vi "Assignment #4 Sarah Bailey.vi"(11 "SCROLLING TEXT":string="LabVIEW VI Assignment ") -> (3 "Array":bool[][](array[boolean])=[[FALSE, FALSE, FALSE, FALSE, TRUE, TRUE, TRUE, FALSE, FALSE, FALSE, FALSE, TRUE, TRUE, TRUE, FALSE, FALSE, FALSE, FALSE, TRUE, TRUE, TRUE, FALSE, FALSE, FALSE, TRUE, TRUE, TRUE, TRUE, TRUE, FALSE, FALSE, FALSE, TRUE, TRUE, TRUE, TRUE, FALSE, FALSE, TRUE, FALSE, FALSE, FALSE, TRUE, FALSE, FALSE, TRUE, FALSE, FALSE, FALSE, TRUE, FALSE, FALSE, TRUE, TRUE, TRUE, TRUE, TRUE, FALSE, FALSE, TRUE, FALSE, FALSE, FALSE, TRUE, FALSE, FALSE, TRUE, TRUE, TRUE], [FALSE, FALSE, FALSE, TRUE, FALSE, FALSE, FALSE, TRUE, FALSE, FALSE, TRUE, FALSE, FALSE, FALSE, TRUE, FALSE, FALSE, TRUE, FALSE, FALSE, FALSE, TRUE, FALSE, FALSE, FALSE, FALSE, TRUE, FALSE, FALSE, FALSE, FALSE, TRUE, FALSE, FALSE, FALSE, FALSE, FALSE, FALSE, TRUE, TRUE, FALSE, FALSE, TRUE, FALSE, FALSE, TRUE, TRUE, FALSE, TRUE, TRUE, FALSE, FALSE, TRUE, FALSE, FALSE, FALSE, FALSE, FALSE, FALSE, TRUE, TRUE, FALSE, FALSE, TRUE, FALSE, FALSE, FALSE, FALSE, TRUE], [FALSE, FALSE, FALSE, TRUE, FALSE, FALSE, FALSE, TRUE, FALSE, FALSE, TRUE, FALSE, FALSE, FALSE, FALSE, FALSE, FALSE, TRUE, FALSE, FALSE, FALSE, FALSE, FALSE, FALSE, FALSE, FALSE, TRUE, FALSE, FALSE, FALSE, FALSE, TRUE, FALSE, FALSE, FALSE, FALSE, FALSE, FALSE, TRUE, FALSE, TRUE, FALSE, TRUE, FALSE, FALSE, TRUE, FALSE, TRUE, FALSE, TRUE, FALSE, FALSE, TRUE, FALSE, FALSE, FALSE, FALSE, FALSE, FALSE, TRUE, FALSE, TRUE, FALSE, TRUE, FALSE, FALSE, FALSE, FALSE, TRUE], [FALSE, FALSE, FALSE, TRUE, TRUE, TRUE, TRUE, TRUE, FALSE, FALSE, FALSE, TRUE, TRUE, TRUE, FALSE, FALSE, FALSE, FALSE, TRUE, TRUE, TRUE, FALSE, FALSE, FALSE, FALSE, FALSE, TRUE, FALSE, FALSE, FALSE, FALSE, TRUE, FALSE, TRUE, TRUE, TRUE, FALSE, FALSE, TRUE, FALSE, TRUE, FALSE, TRUE, FALSE, FALSE, TRUE, FALSE, TRUE, FALSE, TRUE, FALSE, FALSE, TRUE, TRUE, TRUE, TRUE, FALSE, FALSE, FALSE, TRUE, FALSE, TRUE, FALSE, TRUE, FALSE, FALSE, FALSE, FALSE, TRUE], [FALSE, FALSE, FALSE, TRUE, FALSE, FALSE, FALSE, TRUE, FALSE, FALSE, FALSE, FALSE, FALSE, FALSE, TRUE, FALSE, FALSE, FALSE, FALSE, FALSE, FALSE, TRUE, FALSE, FALSE, FALSE, FALSE, TRUE, FALSE, FALSE, FALSE, FALSE, TRUE, FALSE, FALSE, FALSE, TRUE, FALSE, FALSE, TRUE, FALSE, FALSE, TRUE, TRUE, FALSE, FALSE, TRUE, FALSE, FALSE, FALSE, TRUE, FALSE, FALSE, TRUE, FALSE, FALSE, FALSE, FALSE, FALSE, FALSE, TRUE, FALSE, FALSE, TRUE, TRUE, FALSE, FALSE, FALSE, FALSE, TRUE], [FALSE, FALSE, FALSE, TRUE, FALSE, FALSE, FALSE, TRUE, FALSE, FALSE, TRUE, FALSE, FALSE, FALSE, TRUE, FALSE, FALSE, TRUE, FALSE, FALSE, FALSE, TRUE, FALSE, FALSE, FALSE, FALSE, TRUE, FALSE, FALSE, FALSE, FALSE, TRUE, FALSE, FALSE, FALSE, TRUE, FALSE, FALSE, TRUE, FALSE, FALSE, FALSE, TRUE, FALSE, FALSE, TRUE, FALSE, FALSE, FALSE, TRUE, FALSE, FALSE, TRUE, FALSE, FALSE, FALSE, FALSE, FALSE, FALSE, TRUE, FALSE, FALSE, FALSE, TRUE, FALSE, FALSE, FALSE, FALSE, TRUE], [FALSE, FALSE, FALSE, TRUE, FALSE, FALSE, FALSE, TRUE, FALSE, FALSE, FALSE, TRUE, TRUE, TRUE, FALSE, FALSE, FALSE, FALSE, TRUE, TRUE, TRUE, FALSE, FALSE, FALSE, TRUE, TRUE, TRUE, TRUE, TRUE, FALSE, FALSE, FALSE, TRUE, TRUE, TRUE, TRUE, FALSE, FALSE, TRUE, FALSE, FALSE, FALSE, TRUE, FALSE, FALSE, TRUE, FALSE, FALSE, FALSE, TRUE, FALSE, FALSE, TRUE, TRUE, TRUE, TRUE, TRUE, FALSE, FALSE, TRUE, FALSE, FALSE, FALSE, TRUE, FALSE, FALSE, FALSE, FALSE, TRUE]])   [LabVIEW 2013]
panel:
  in  "stop":bool
  in  "SPEED":dbl(slide)=73.25102880658436 scale=0.0..200.0
  # "FASTER"
  # "SLOWER"
  # "Developed by: Sarah Bailey\nEngineering Applications Lab\nSummer 2014\nAssignment #4\nWorked with: Alexander Offredi and Clair Cunningham"
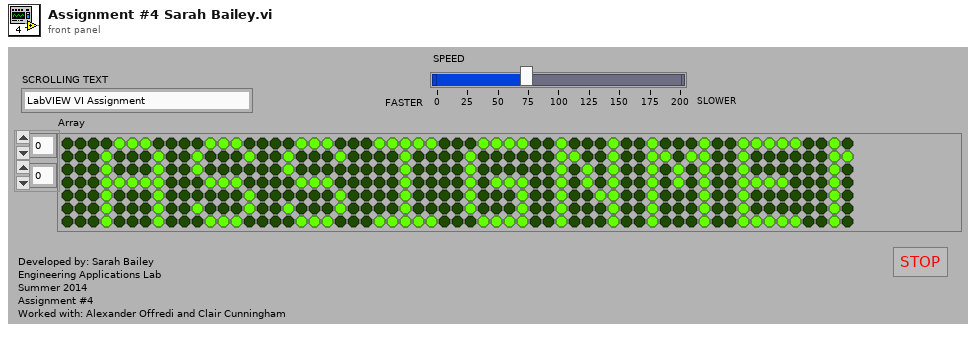
[diagram p1: front panel]
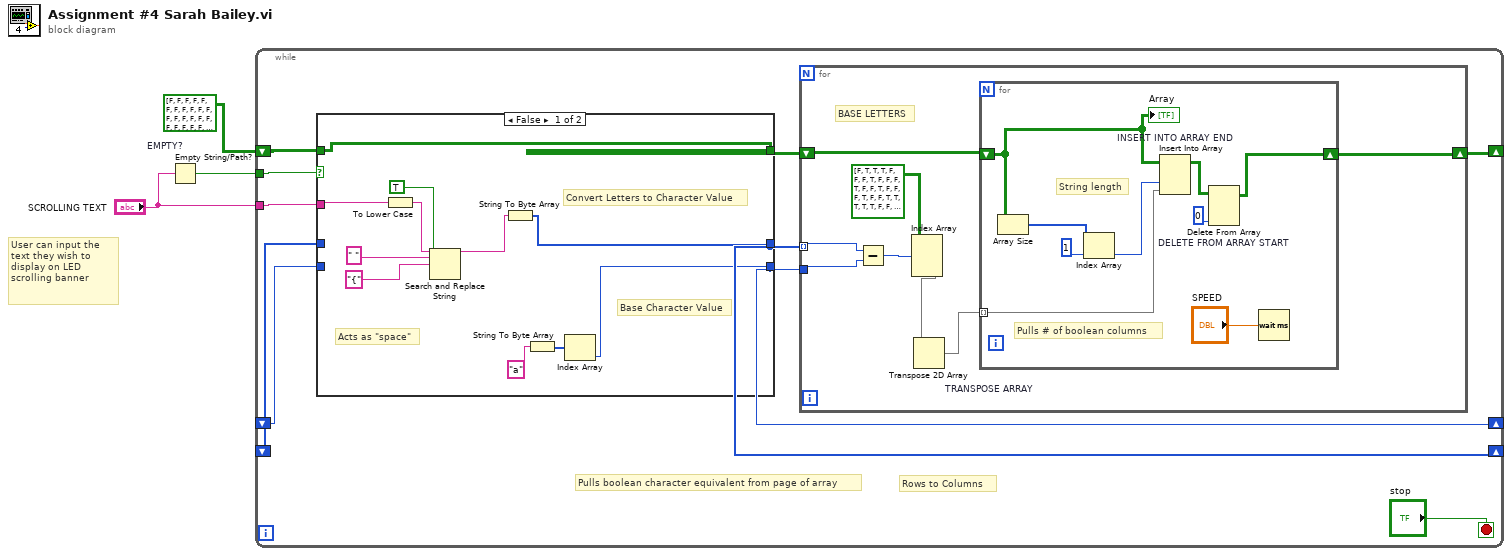
[diagram p0: block diagram]
diagram:
  # "User can input the text they wish to display on LED scrolling banner"
  n1 = Empty String/Path? "EMPTY?"(string/path="SCROLLING TEXT") -> (empty?=w2:bool)
  n2 = while {
    tunnel: "SCROLLING TEXT" -> [w13]
    tunnel: w2 -> [w12]
    shift-right: [w5] -> _
    shift-left: bool[][] [[FALSE, FALSE, FALSE, FALSE, FALSE, FALSE, FALSE, FALSE, FALSE, FALSE, FALSE, FALSE, FALSE, FALSE, FALSE, FALSE, FALSE, FALSE, FALSE, FALSE, FALSE, FALSE, FALSE, FALSE, FALSE, FALSE, FALSE, FALSE, FALSE, FALSE, FALSE, FALSE, FALSE, FALSE, FALSE, FALSE, FALSE, FALSE, FALSE, FALSE, FALSE, FALSE, FALSE, FALSE, FALSE, FALSE, FALSE, FALSE, FALSE, FALSE, FALSE, FALSE, FALSE, FALSE, FALSE, FALSE, FALSE, FALSE, FALSE, FALSE, FALSE, FALSE, FALSE, FALSE, FALSE, FALSE, FALSE, FALSE, FALSE], [FALSE, FALSE, FALSE, FALSE, FALSE, FALSE, FALSE, FALSE, FALSE, FALSE, FALSE, FALSE, FALSE, FALSE, FALSE, FALSE, FALSE, FALSE, FALSE, FALSE, FALSE, FALSE, FALSE, FALSE, FALSE, FALSE, FALSE, FALSE, FALSE, FALSE, FALSE, FALSE, FALSE, FALSE, FALSE, FALSE, FALSE, FALSE, FALSE, FALSE, FALSE, FALSE, FALSE, FALSE, FALSE, FALSE, FALSE, FALSE, FALSE, FALSE, FALSE, FALSE, FALSE, FALSE, FALSE, FALSE, FALSE, FALSE, FALSE, FALSE, FALSE, FALSE, FALSE, FALSE, FALSE, FALSE, FALSE, FALSE, FALSE], [FALSE, FALSE, FALSE, FALSE, FALSE, FALSE, FALSE, FALSE, FALSE, FALSE, FALSE, FALSE, FALSE, FALSE, FALSE, FALSE, FALSE, FALSE, FALSE, FALSE, FALSE, FALSE, FALSE, FALSE, FALSE, FALSE, FALSE, FALSE, FALSE, FALSE, FALSE, FALSE, FALSE, FALSE, FALSE, FALSE, FALSE, FALSE, FALSE, FALSE, FALSE, FALSE, FALSE, FALSE, FALSE, FALSE, FALSE, FALSE, FALSE, FALSE, FALSE, FALSE, FALSE, FALSE, FALSE, FALSE, FALSE, FALSE, FALSE, FALSE, FALSE, FALSE, FALSE, FALSE, FALSE, FALSE, FALSE, FALSE, FALSE], [FALSE, FALSE, FALSE, FALSE, FALSE, FALSE, FALSE, FALSE, FALSE, FALSE, FALSE, FALSE, FALSE, FALSE, FALSE, FALSE, FALSE, FALSE, FALSE, FALSE, FALSE, FALSE, FALSE, FALSE, FALSE, FALSE, FALSE, FALSE, FALSE, FALSE, FALSE, FALSE, FALSE, FALSE, FALSE, FALSE, FALSE, FALSE, FALSE, FALSE, FALSE, FALSE, FALSE, FALSE, FALSE, FALSE, FALSE, FALSE, FALSE, FALSE, FALSE, FALSE, FALSE, FALSE, FALSE, FALSE, FALSE, FALSE, FALSE, FALSE, FALSE, FALSE, FALSE, FALSE, FALSE, FALSE, FALSE, FALSE, FALSE], [FALSE, FALSE, FALSE, FALSE, FALSE, FALSE, FALSE, FALSE, FALSE, FALSE, FALSE, FALSE, FALSE, FALSE, FALSE, FALSE, FALSE, FALSE, FALSE, FALSE, FALSE, FALSE, FALSE, FALSE, FALSE, FALSE, FALSE, FALSE, FALSE, FALSE, FALSE, FALSE, FALSE, FALSE, FALSE, FALSE, FALSE, FALSE, FALSE, FALSE, FALSE, FALSE, FALSE, FALSE, FALSE, FALSE, FALSE, FALSE, FALSE, FALSE, FALSE, FALSE, FALSE, FALSE, FALSE, FALSE, FALSE, FALSE, FALSE, FALSE, FALSE, FALSE, FALSE, FALSE, FALSE, FALSE, FALSE, FALSE, FALSE], [FALSE, FALSE, FALSE, FALSE, FALSE, FALSE, FALSE, FALSE, FALSE, FALSE, FALSE, FALSE, FALSE, FALSE, FALSE, FALSE, FALSE, FALSE, FALSE, FALSE, FALSE, FALSE, FALSE, FALSE, FALSE, FALSE, FALSE, FALSE, FALSE, FALSE, FALSE, FALSE, FALSE, FALSE, FALSE, FALSE, FALSE, FALSE, FALSE, FALSE, FALSE, FALSE, FALSE, FALSE, FALSE, FALSE, FALSE, FALSE, FALSE, FALSE, FALSE, FALSE, FALSE, FALSE, FALSE, FALSE, FALSE, FALSE, FALSE, FALSE, FALSE, FALSE, FALSE, FALSE, FALSE, FALSE, FALSE, FALSE, FALSE], [FALSE, FALSE, FALSE, FALSE, FALSE, FALSE, FALSE, FALSE, FALSE, FALSE, FALSE, FALSE, FALSE, FALSE, FALSE, FALSE, FALSE, FALSE, FALSE, FALSE, FALSE, FALSE, FALSE, FALSE, FALSE, FALSE, FALSE, FALSE, FALSE, FALSE, FALSE, FALSE, FALSE, FALSE, FALSE, FALSE, FALSE, FALSE, FALSE, FALSE, FALSE, FALSE, FALSE, FALSE, FALSE, FALSE, FALSE, FALSE, FALSE, FALSE, FALSE, FALSE, FALSE, FALSE, FALSE, FALSE, FALSE, FALSE, FALSE, FALSE, FALSE, FALSE, FALSE, FALSE, FALSE, FALSE, FALSE, FALSE, FALSE]] ("Array 2") -> [w10]
    shift-right: [w9] -> _
    shift-left: _ -> [w7]
    shift-right: [w8] -> _
    shift-left: _ -> [w6]
    stop <- "stop" stop-if-true
    # "Rows to Columns"
    # "Pulls boolean character equivalent from page of array"
    n3 = case shown="False" w12 {
      tunnel: [w14 w26] -> w9
      tunnel: [w22 w25] -> w8
      tunnel: w13 -> [w21 _]
      tunnel: [w15 w27] -> w11
      tunnel: w10 -> [w15 w27]
      tunnel: w7 -> [_ w26]
      tunnel: w6 -> [_ w25]
      frame False {
        # "Base Character Value"
        # "Convert Letters to Character Value"
        # "Acts as \"space\""
        n4 = To Lower Case(string=w21) -> (all lower case string=w16:string)
        n5 = Search and Replace String(replace all?=TRUE ("replace all? (F)"), input string=w16, search string=" ", replace string="{") -> (result string=w19:string)  [unwired: 4 in, 3 out]
        n6 = String To Byte Array(string=w19) -> (unsigned byte array=w14:u8[])
        n7 = String To Byte Array(string="a") -> (unsigned byte array=w23:u8[])
        n8 = Index Array "INDEX ARRAY"(array=w23) -> (element=w22:u8)  [unwired: 1 in]
      }
      frame True {
      }
    }
    n9 = for {
      shift-right: [w31] -> w5
      shift-left: w11 -> [w28]
      tunnel: w9 -> [w35] mode=indexing
      tunnel: w8 -> [w34]
      # "BASE LETTERS"
      n10 = Subtract(x=w35, y=w34) -> (x-y=w32:u8)
      n11 = Index Array "INDEX ARRAY"(array=bool[][][] [[[FALSE, TRUE, TRUE, TRUE, FALSE, FALSE, FALSE], [TRUE, FALSE, FALSE, FALSE, TRUE, FALSE, FALSE], [TRUE, FALSE, FALSE, FALSE, TRUE, FALSE, FALSE], [TRUE, TRUE, TRUE, TRUE, TRUE, FALSE, FALSE], [TRUE, FALSE, FALSE, FALSE, TRUE, FALSE, FALSE], [TRUE, FALSE, FALSE, FALSE, TRUE, FALSE, FALSE], [TRUE, FALSE, FALSE, FALSE, TRUE, FALSE, FALSE]], [[TRUE, TRUE, TRUE, TRUE, FALSE, FALSE, FALSE], [TRUE, FALSE, FALSE, FALSE, TRUE, FALSE, FALSE], [TRUE, FALSE, FALSE, FALSE, TRUE, FALSE, FALSE], [TRUE, TRUE, TRUE, TRUE, FALSE, FALSE, FALSE], [TRUE, FALSE, FALSE, FALSE, TRUE, FALSE, FALSE], [TRUE, FALSE, FALSE, FALSE, TRUE, FALSE, FALSE], [TRUE, TRUE, TRUE, TRUE, TRUE, FALSE, FALSE]], [[FALSE, TRUE, TRUE, TRUE, TRUE, FALSE, FALSE], [TRUE, FALSE, FALSE, FALSE, FALSE, FALSE, FALSE], [TRUE, FALSE, FALSE, FALSE, FALSE, FALSE, FALSE], [TRUE, FALSE, FALSE, FALSE, FALSE, FALSE, FALSE], [TRUE, FALSE, FALSE, FALSE, FALSE, FALSE, FALSE], [TRUE, FALSE, FALSE, FALSE, FALSE, FALSE, FALSE], [FALSE, TRUE, TRUE, TRUE, TRUE, FALSE, FALSE]], [[TRUE, TRUE, TRUE, FALSE, FALSE, FALSE, FALSE], [TRUE, FALSE, FALSE, TRUE, FALSE, FALSE, FALSE], [TRUE, FALSE, FALSE, FALSE, TRUE, FALSE, FALSE], [TRUE, FALSE, FALSE, FALSE, TRUE, FALSE, FALSE], [TRUE, FALSE, FALSE, FALSE, TRUE, FALSE, FALSE], [TRUE, FALSE, FALSE, TRUE, FALSE, FALSE, FALSE], [TRUE, TRUE, TRUE, FALSE, FALSE, FALSE, FALSE]], [[TRUE, TRUE, TRUE, TRUE, TRUE, FALSE, FALSE], [TRUE, FALSE, FALSE, FALSE, FALSE, FALSE, FALSE], [TRUE, FALSE, FALSE, FALSE, FALSE, FALSE, FALSE], [TRUE, TRUE, TRUE, TRUE, FALSE, FALSE, FALSE], [TRUE, FALSE, FALSE, FALSE, FALSE, FALSE, FALSE], [TRUE, FALSE, FALSE, FALSE, FALSE, FALSE, FALSE], [TRUE, TRUE, TRUE, TRUE, TRUE, FALSE, FALSE]], [[TRUE, TRUE, TRUE, TRUE, TRUE, FALSE, FALSE], [TRUE, FALSE, FALSE, FALSE, FALSE, FALSE, FALSE], [TRUE, FALSE, FALSE, FALSE, FALSE, FALSE, FALSE], [TRUE, TRUE, TRUE, TRUE, FALSE, FALSE, FALSE], [TRUE, FALSE, FALSE, FALSE, FALSE, FALSE, FALSE], [TRUE, FALSE, FALSE, FALSE, FALSE, FALSE, FALSE], [TRUE, FALSE, FALSE, FALSE, FALSE, FALSE, FALSE]], [[FALSE, TRUE, TRUE, TRUE, TRUE, FALSE, FALSE], [TRUE, FALSE, FALSE, FALSE, FALSE, FALSE, FALSE], [TRUE, FALSE, FALSE, FALSE, FALSE, FALSE, FALSE], [TRUE, FALSE, TRUE, TRUE, TRUE, FALSE, FALSE], [TRUE, FALSE, FALSE, FALSE, TRUE, FALSE, FALSE], [TRUE, FALSE, FALSE, FALSE, TRUE, FALSE, FALSE], [FALSE, TRUE, TRUE, TRUE, TRUE, FALSE, FALSE]], [[TRUE, FALSE, FALSE, FALSE, TRUE, FALSE, FALSE], [TRUE, FALSE, FALSE, FALSE, TRUE, FALSE, FALSE], [TRUE, FALSE, FALSE, FALSE, TRUE, FALSE, FALSE], [TRUE, TRUE, TRUE, TRUE, TRUE, FALSE, FALSE], [TRUE, FALSE, FALSE, FALSE, TRUE, FALSE, FALSE], [TRUE, FALSE, FALSE, FALSE, TRUE, FALSE, FALSE], [TRUE, FALSE, FALSE, FALSE, TRUE, FALSE, FALSE]], [[TRUE, TRUE, TRUE, TRUE, TRUE, FALSE, FALSE], [FALSE, FALSE, TRUE, FALSE, FALSE, FALSE, FALSE], [FALSE, FALSE, TRUE, FALSE, FALSE, FALSE, FALSE], [FALSE, FALSE, TRUE, FALSE, FALSE, FALSE, FALSE], [FALSE, FALSE, TRUE, FALSE, FALSE, FALSE, FALSE], [FALSE, FALSE, TRUE, FALSE, FALSE, FALSE, FALSE], [TRUE, TRUE, TRUE, TRUE, TRUE, FALSE, FALSE]], [[TRUE, TRUE, TRUE, TRUE, TRUE, FALSE, FALSE], [FALSE, FALSE, TRUE, FALSE, FALSE, FALSE, FALSE], [FALSE, FALSE, TRUE, FALSE, FALSE, FALSE, FALSE], [FALSE, FALSE, TRUE, FALSE, FALSE, FALSE, FALSE], [TRUE, FALSE, TRUE, FALSE, FALSE, FALSE, FALSE], [TRUE, FALSE, TRUE, FALSE, FALSE, FALSE, FALSE], [TRUE, TRUE, TRUE, FALSE, FALSE, FALSE, FALSE]], [[TRUE, FALSE, FALSE, FALSE, TRUE, FALSE, FALSE], [TRUE, FALSE, FALSE, TRUE, FALSE, FALSE, FALSE], [TRUE, FALSE, TRUE, FALSE, FALSE, FALSE, FALSE], [TRUE, TRUE, FALSE, FALSE, FALSE, FALSE, FALSE], [TRUE, FALSE, TRUE, FALSE, FALSE, FALSE, FALSE], [TRUE, FALSE, FALSE, TRUE, FALSE, FALSE, FALSE], [TRUE, FALSE, FALSE, FALSE, TRUE, FALSE, FALSE]], [[TRUE, FALSE, FALSE, FALSE, FALSE, FALSE, FALSE], [TRUE, FALSE, FALSE, FALSE, FALSE, FALSE, FALSE], [TRUE, FALSE, FALSE, FALSE, FALSE, FALSE, FALSE], [TRUE, FALSE, FALSE, FALSE, FALSE, FALSE, FALSE], [TRUE, FALSE, FALSE, FALSE, FALSE, FALSE, FALSE], [TRUE, FALSE, FALSE, FALSE, FALSE, FALSE, FALSE], [TRUE, TRUE, TRUE, TRUE, TRUE, FALSE, FALSE]], [[TRUE, FALSE, FALSE, FALSE, TRUE, FALSE, FALSE], [TRUE, TRUE, FALSE, TRUE, TRUE, FALSE, FALSE], [TRUE, FALSE, TRUE, FALSE, TRUE, FALSE, FALSE], [TRUE, FALSE, TRUE, FALSE, TRUE, FALSE, FALSE], [TRUE, FALSE, FALSE, FALSE, TRUE, FALSE, FALSE], [TRUE, FALSE, FALSE, FALSE, TRUE, FALSE, FALSE], [TRUE, FALSE, FALSE, FALSE, TRUE, FALSE, FALSE]], [[TRUE, FALSE, FALSE, FALSE, TRUE, FALSE, FALSE], [TRUE, TRUE, FALSE, FALSE, TRUE, FALSE, FALSE], [TRUE, FALSE, TRUE, FALSE, TRUE, FALSE, FALSE], [TRUE, FALSE, TRUE, FALSE, TRUE, FALSE, FALSE], [TRUE, FALSE, FALSE, TRUE, TRUE, FALSE, FALSE], [TRUE, FALSE, FALSE, FALSE, TRUE, FALSE, FALSE], [TRUE, FALSE, FALSE, FALSE, TRUE, FALSE, FALSE]], [[FALSE, TRUE, TRUE, TRUE, FALSE, FALSE, FALSE], [TRUE, FALSE, FALSE, FALSE, TRUE, FALSE, FALSE], [TRUE, FALSE, FALSE, FALSE, TRUE, FALSE, FALSE], [TRUE, FALSE, FALSE, FALSE, TRUE, FALSE, FALSE], [TRUE, FALSE, FALSE, FALSE, TRUE, FALSE, FALSE], [TRUE, FALSE, FALSE, FALSE, TRUE, FALSE, FALSE], [FALSE, TRUE, TRUE, TRUE, FALSE, FALSE, FALSE]], [[TRUE, TRUE, TRUE, TRUE, FALSE, FALSE, FALSE], [TRUE, FALSE, FALSE, FALSE, TRUE, FALSE, FALSE], [TRUE, FALSE, FALSE, FALSE, TRUE, FALSE, FALSE], [TRUE, TRUE, TRUE, TRUE, FALSE, FALSE, FALSE], [TRUE, FALSE, FALSE, FALSE, FALSE, FALSE, FALSE], [TRUE, FALSE, FALSE, FALSE, FALSE, FALSE, FALSE], [TRUE, FALSE, FALSE, FALSE, FALSE, FALSE, FALSE]], [[FALSE, TRUE, TRUE, TRUE, FALSE, FALSE, FALSE], [TRUE, FALSE, FALSE, FALSE, TRUE, FALSE, FALSE], [TRUE, FALSE, FALSE, FALSE, TRUE, FALSE, FALSE], [TRUE, FALSE, TRUE, FALSE, TRUE, FALSE, FALSE], [TRUE, FALSE, TRUE, FALSE, TRUE, FALSE, FALSE], [TRUE, FALSE, FALSE, TRUE, FALSE, FALSE, FALSE], [FALSE, TRUE, TRUE, FALSE, TRUE, FALSE, FALSE]], [[TRUE, TRUE, TRUE, TRUE, FALSE, FALSE, FALSE], [TRUE, FALSE, FALSE, FALSE, TRUE, FALSE, FALSE], [TRUE, FALSE, FALSE, FALSE, TRUE, FALSE, FALSE], [TRUE, TRUE, TRUE, TRUE, FALSE, FALSE, FALSE], [TRUE, FALSE, TRUE, FALSE, FALSE, FALSE, FALSE], [TRUE, FALSE, FALSE, TRUE, FALSE, FALSE, FALSE], [TRUE, FALSE, FALSE, FALSE, TRUE, FALSE, FALSE]], [[FALSE, TRUE, TRUE, TRUE, FALSE, FALSE, FALSE], [TRUE, FALSE, FALSE, FALSE, TRUE, FALSE, FALSE], [TRUE, FALSE, FALSE, FALSE, FALSE, FALSE, FALSE], [FALSE, TRUE, TRUE, TRUE, FALSE, FALSE, FALSE], [FALSE, FALSE, FALSE, FALSE, TRUE, FALSE, FALSE], [TRUE, FALSE, FALSE, FALSE, TRUE, FALSE, FALSE], [FALSE, TRUE, TRUE, TRUE, FALSE, FALSE, FALSE]], [[TRUE, TRUE, TRUE, TRUE, TRUE, FALSE, FALSE], [FALSE, FALSE, TRUE, FALSE, FALSE, FALSE, FALSE], [FALSE, FALSE, TRUE, FALSE, FALSE, FALSE, FALSE], [FALSE, FALSE, TRUE, FALSE, FALSE, FALSE, FALSE], [FALSE, FALSE, TRUE, FALSE, FALSE, FALSE, FALSE], [FALSE, FALSE, TRUE, FALSE, FALSE, FALSE, FALSE], [FALSE, FALSE, TRUE, FALSE, FALSE, FALSE, FALSE]], [[TRUE, FALSE, FALSE, FALSE, TRUE, FALSE, FALSE], [TRUE, FALSE, FALSE, FALSE, TRUE, FALSE, FALSE], [TRUE, FALSE, FALSE, FALSE, TRUE, FALSE, FALSE], [TRUE, FALSE, FALSE, FALSE, TRUE, FALSE, FALSE], [TRUE, FALSE, FALSE, FALSE, TRUE, FALSE, FALSE], [TRUE, FALSE, FALSE, FALSE, TRUE, FALSE, FALSE], [FALSE, TRUE, TRUE, TRUE, FALSE, FALSE, FALSE]], [[TRUE, FALSE, FALSE, FALSE, TRUE, FALSE, FALSE], [TRUE, FALSE, FALSE, FALSE, TRUE, FALSE, FALSE], [TRUE, FALSE, FALSE, FALSE, TRUE, FALSE, FALSE], [TRUE, FALSE, FALSE, FALSE, TRUE, FALSE, FALSE], [TRUE, FALSE, FALSE, FALSE, TRUE, FALSE, FALSE], [FALSE, TRUE, FALSE, TRUE, FALSE, FALSE, FALSE], [FALSE, FALSE, TRUE, FALSE, FALSE, FALSE, FALSE]], [[TRUE, FALSE, FALSE, FALSE, TRUE, FALSE, FALSE], [TRUE, FALSE, FALSE, FALSE, TRUE, FALSE, FALSE], [TRUE, FALSE, FALSE, FALSE, TRUE, FALSE, FALSE], [TRUE, FALSE, FALSE, FALSE, TRUE, FALSE, FALSE], [TRUE, FALSE, TRUE, FALSE, TRUE, FALSE, FALSE], [TRUE, TRUE, FALSE, TRUE, TRUE, FALSE, FALSE], [TRUE, FALSE, FALSE, FALSE, TRUE, FALSE, FALSE]], [[TRUE, FALSE, FALSE, FALSE, TRUE, FALSE, FALSE], [FALSE, TRUE, FALSE, TRUE, FALSE, FALSE, FALSE], [FALSE, TRUE, FALSE, TRUE, FALSE, FALSE, FALSE], [FALSE, FALSE, TRUE, FALSE, FALSE, FALSE, FALSE], [FALSE, TRUE, FALSE, TRUE, FALSE, FALSE, FALSE], [FALSE, TRUE, FALSE, TRUE, FALSE, FALSE, FALSE], [TRUE, FALSE, FALSE, FALSE, TRUE, FALSE, FALSE]], [[TRUE, FALSE, FALSE, FALSE, TRUE, FALSE, FALSE], [TRUE, FALSE, FALSE, FALSE, TRUE, FALSE, FALSE], [FALSE, TRUE, FALSE, TRUE, FALSE, FALSE, FALSE], [FALSE, FALSE, TRUE, FALSE, FALSE, FALSE, FALSE], [FALSE, FALSE, TRUE, FALSE, FALSE, FALSE, FALSE], [FALSE, FALSE, TRUE, FALSE, FALSE, FALSE, FALSE], [FALSE, FALSE, TRUE, FALSE, FALSE, FALSE, FALSE]], [[TRUE, TRUE, TRUE, TRUE, TRUE, FALSE, FALSE], [FALSE, FALSE, FALSE, TRUE, FALSE, FALSE, FALSE], [FALSE, FALSE, TRUE, FALSE, FALSE, FALSE, FALSE], [FALSE, FALSE, TRUE, FALSE, FALSE, FALSE, FALSE], [FALSE, TRUE, FALSE, FALSE, FALSE, FALSE, FALSE], [TRUE, FALSE, FALSE, FALSE, FALSE, FALSE, FALSE], [TRUE, TRUE, TRUE, TRUE, TRUE, FALSE, FALSE]], [[FALSE, FALSE, FALSE, FALSE, FALSE, FALSE, FALSE], [FALSE, FALSE, FALSE, FALSE, FALSE, FALSE, FALSE], [FALSE, FALSE, FALSE, FALSE, FALSE, FALSE, FALSE], [FALSE, FALSE, FALSE, FALSE, FALSE, FALSE, FALSE], [FALSE, FALSE, FALSE, FALSE, FALSE, FALSE, FALSE], [FALSE, FALSE, FALSE, FALSE, FALSE, FALSE, FALSE], [FALSE, FALSE, FALSE, FALSE, FALSE, FALSE, FALSE]]] ("Array 2"), index (dim 0)=w32) -> (element=w30:bool[][])  [unwired: 2 in]
      n12 = Transpose 2D Array "TRANSPOSE ARRAY"(2D array=w30) -> (transposed array=w29:bool[][])
      n13 = for {
        shift-right: [w38] -> w31
        shift-left: w28 -> [w37]
        tunnel: w29 -> [w44] mode=indexing
        # "Pulls # of boolean columns"
        # "String length"
        n14 = Array Size(array=w37) -> (size(s)=w43:i32[])
        n15 = Index Array "INDEX ARRAY"(array=w43, index=1 ("Index")) -> (element=w41:i32)
        n16 = Insert Into Array "INSERT INTO ARRAY END"(array=w37, index (col)=w41, new element=w44) -> (w40:bool[][])  [unwired: 1 in]
        n17 = Delete From Array "DELETE FROM ARRAY START"(array=w40, index (col)=0 ("Disabled Index (col)")) -> (array with subset deleted=w38:bool[][])  [unwired: 2 in, 1 out]
        n18 = Wait (ms)(milliseconds to wait="SPEED") -> ()  [unwired: 1 out]
        "Array" <- w37
      }
    }
  }
